vi "AMC e.bloxx Get Device Identification.vi"(8 "error in (no error)":errorcluster, 10 "Module Address":i32, 11 "VISA Resource Name":refnum<visa-resource-name>) -> (0 "error out":errorcluster, 1 "Model Name":string, 2 "Vendor Name":string, 3 "VISA Resource Name out":refnum<visa-resource-name>, 4 "Software Revision":string, 5 "Hardware Revision":string)   [LabVIEW 2013]
doc: "<B>AMC - Analytik & Messtechnik GmbH Chemnitz</B>\n\nLabVIEW Drivers for e.bloxx series from Gantner Instruments\n\nThis VI reads the device identification from the module specified by <B>Module Address</B>."
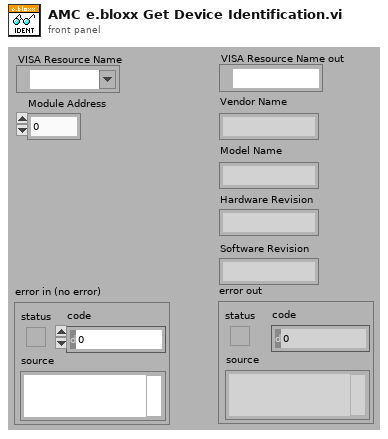
[diagram p1: front panel]
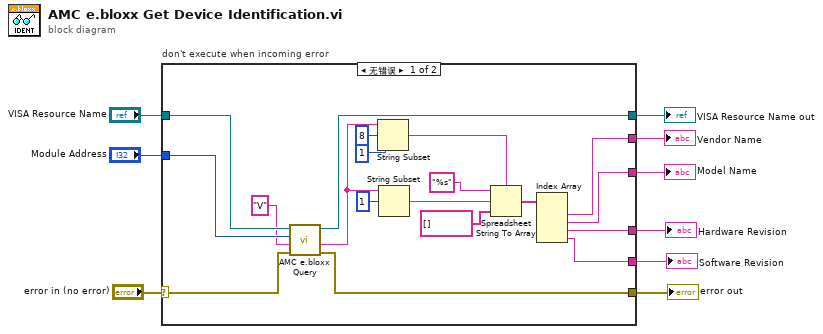
[diagram p0: block diagram]
diagram:
  n1 = case "don't execute when incoming error" shown="无错误" "error in (no error)" {
    selector: "error in (no error)" -> [w28 w30]
    tunnel: [w24 w30] -> w8
    tunnel: "VISA Resource Name" -> [w26 w29]
    tunnel: "Module Address" -> [w27 _]
    tunnel: [w14 w29] -> w5
    tunnel: [w18 _] -> w4
    tunnel: [w17 _] -> w3
    tunnel: [w16 _] -> w2
    tunnel: [w15 _] -> w1
    frame No Error {
      n2 = call "AMC e.bloxx Query.vi"("error in (no error)"=w28, "Module Command"="V", "Module Address"=w27, "VISA Resource Name"=w26) -> ("error out"=w24:errorcluster, "Module Response"=w13:string, "VISA Resource Name out"=w14:refnum<visa-resource-name>)  [unwired: 5 in]
      n3 = String Subset(string=w13, offset (0)=8, length (rest)=1 ("length (rest)")) -> (substring=w10:string)
      n4 = String Subset(string=w13, offset (0)=1) -> (substring=w20:string)  [unwired: 1 in]
      n5 = Spreadsheet String To Array(delimiter (Tab)=w10, format string="%s", spreadsheet string=w20, array type (2D Dbl)=string[] []) -> (array=w19:string[])
      n6 = Index Array(array=w19) -> (element #1=w18:string, element #2=w17:string, element #3=w16:string, element #4=w15:string)  [unwired: 4 in]
    }
    frame Error {
    }
  }
  "error out" <- w8
  "VISA Resource Name out" <- w5
  "Vendor Name" <- w4
  "Model Name" <- w3
  "Hardware Revision" <- w2
  "Software Revision" <- w1
